vi "LCD(SubVI).vi"(8 "error in (no error)":errorcluster, 10 "Data":i8[](array[numeric]), 11 "LINX Resource in":T1) -> (0 "error out":errorcluster, 1 "LINX Resource out":T1, 2 "Response":u8[](array[numeric]), 3 "string":string, 5 "string 2":string)   [LabVIEW 2020]
uses:
  <vilib>/MakerHub/LINX/Private/Type Defs/LINX Ref.ctl
  <vilib>/MakerHub/LINX/Private/Type Defs/Platform.ctl
  <vilib>/MakerHub/LINX/Private/Type Defs/Interface.ctl
  <vilib>/MakerHub/LINX/Private/Device/Type Defs/LINX Device Config.ctl
  <vilib>/MakerHub/LINX/Private/Device/Type Defs/TCP Config.ctl
  <vilib>/MakerHub/LINX/Private/Device/Type Defs/Channels.ctl
  <vilib>/MakerHub/LINX/LMH-LINX.lvlib
  <vilib>/MakerHub/LINX/Private/Device/Device.lvlib
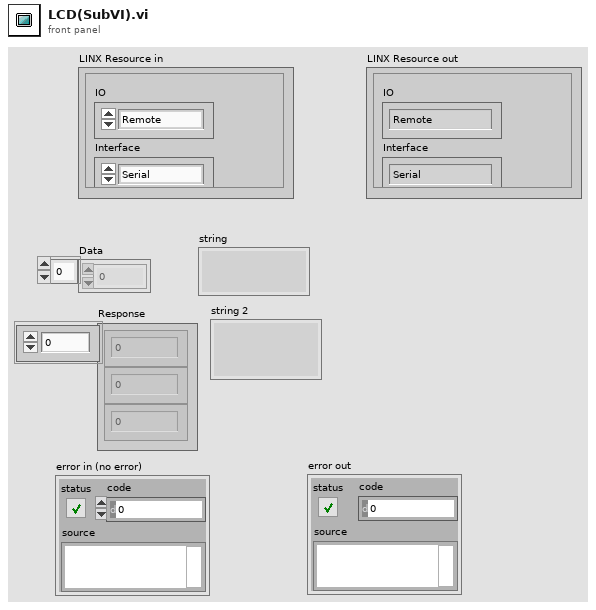
[diagram p1: front panel]
types:
  T1 = typedef "LMH-LINX.lvlib/LINX Ref.ctl" = cluster{"IO":T2, "Interface":T3, "LINX Device Config":T4}
  T2 = typedef "LMH-LINX.lvlib/Platform.ctl" = enum16{"Remote", "Local"}
  T3 = typedef "LMH-LINX.lvlib/Interface.ctl" = enum16{"Serial", "TCP"}
  T4 = typedef "LMH-LINX.lvlib/Device.lvlib/LINX Device Config.ctl" = cluster{"Interface":T3, "COM Port":refnum<visa-resource-name>, "TCP Configuration":T5, "Device Family":u8, "Device ID":u8, "Device Name":string, "TCP Ref":refnum<k5>, "Channels":T6}
  T5 = typedef "LMH-LINX.lvlib/Device.lvlib/TCP Config.ctl" = cluster{"IP Address":string, "Port":u16}
  T6 = typedef "LMH-LINX.lvlib/Channels.ctl" = cluster{"DI":u8[], "DO":u8[], "AI":u8[], "AO":u8[], "PWM":u8[], "QE":u8[], "UART":u8[], "I2C 2":u8[], "SPI":u8[], "CAN":u8[], "Servo":u8[], "AI Ref (V)":dbl, "AI Resolution (Bits)":u8, "AO Ref (V)":dbl, "AO Resolution (Bits)":u8}
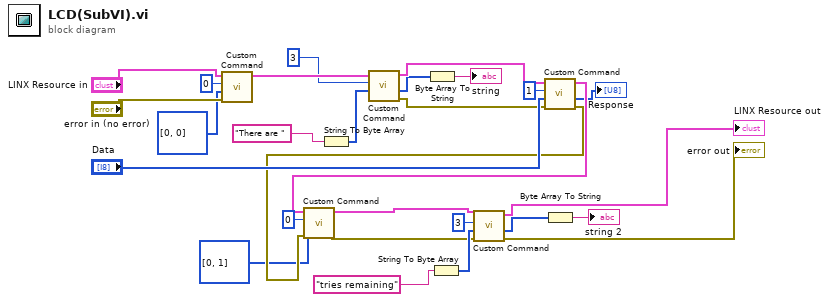
[diagram p0: block diagram]
diagram:
  n1 = call <vilib>:"Custom Command.vi"("Error In"="error in (no error)", "Data"=u8[] [0, 0], "Custom Command Number"=u16 0, "LINX Resource"="LINX Resource in") -> ("LINX Resource"=w6:T1)  [unwired: 4 in, 3 out]
  n2 = String To Byte Array(string="There are " ("String")) -> (unsigned byte array=w8:u8[])
  n3 = call <vilib>:"Custom Command.vi"("Data"=w8, "Custom Command Number"=u16 3, "LINX Resource"=w6) -> ("Error Out"=w12:errorcluster, "Response"=w9:u8[], "LINX Resource"=w11:T1)  [unwired: 5 in, 1 out]
  n4 = Byte Array To String(unsigned byte array=w9) -> (string=→"string":string)
  n5 = String To Byte Array(string="tries remaining" ("String 2")) -> (unsigned byte array=w23:u8[])
  n6 = call <vilib>:"Custom Command.vi"("Error In"=w12, "Data"="Data", "Custom Command Number"=u16 1, "LINX Resource"=w11) -> ("Error Out"=w18:errorcluster, "Response"=→"Response":u8[], "LINX Resource"=w15:T1)  [unwired: 4 in, 1 out]
  n7 = call <vilib>:"Custom Command.vi"("Error In"=w18, "Data"=u8[] [0, 1], "Custom Command Number"=u16 0, "LINX Resource"=w15) -> ("Error Out"=w21:errorcluster, "LINX Resource"=w20:T1)  [unwired: 4 in, 2 out]
  n8 = call <vilib>:"Custom Command.vi"("Error In"=w21, "Data"=w23, "Custom Command Number"=u16 3, "LINX Resource"=w20) -> ("Error Out"=→"error out":errorcluster, "Response"=w24:u8[], "LINX Resource"=→"LINX Resource out":T1)  [unwired: 4 in, 1 out]
  n9 = Byte Array To String(unsigned byte array=w24) -> (string=→"string 2":string)
